vi "CoordinateConvert_ArmToCartesian.vi"(2 "Radius (in)":dbl, 3 "Angle (rad)":dbl) -> (0 "Y (in)":dbl, 1 "X (in)":dbl)   [LabVIEW 2017]
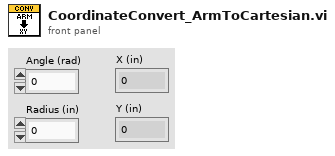
[diagram p1: front panel]
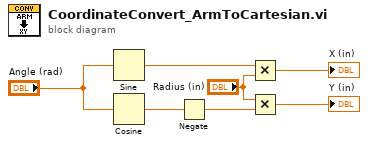
[diagram p0: block diagram]
diagram:
  n1 = Sine(x="Angle (rad)") -> (sin(x)=w7:dbl)
  n2 = Cosine(x="Angle (rad)") -> (cos(x)=w3:dbl)
  n3 = Negate(x=w3) -> (-x=w2:dbl)
  n4 = Multiply(x=w7, y="Radius (in)") -> (x*y=→"X (in)":dbl)
  n5 = Multiply(x="Radius (in)", y=w2) -> (x*y=→"Y (in)":dbl)
